vi "Teleop.vi"(10 "Match Info":T1={"Autonomous Elapsed Seconds"=0.0, "TeleOp Elapsed Seconds"=0.0, "Disabled Elapsed Seconds"=0.0, "Visited Autonomous"=FALSE, "Visited TeleOp"=FALSE, "Visited Disabled"=FALSE, "Autonomous Settings"={"Autonomous Style"=enum."Independent", "VI Refnum"=refnum}}, 11 "Call Context":T2) -> ()   [LabVIEW 2019]
doc: "This VI is called for each enabled TeleOp packet received from the DS. It is typically used to read from joysticks and other inputs and update I/O or setpoints for timed control loops. It should complete and return within 20 milliseconds or risk missing DS packets."
uses:
  <vilib>/Rock Robotics/WPI/DriverStation/WPI_DriverStationDerivedRobotMode.ctl
  <vilib>/Rock Robotics/WPI/DriverStation/WPI_DriverStationMatch Info.ctl
  <vilib>/Rock Robotics/WPI/Utilities/WPI_GetSetVariantRefNum.vi
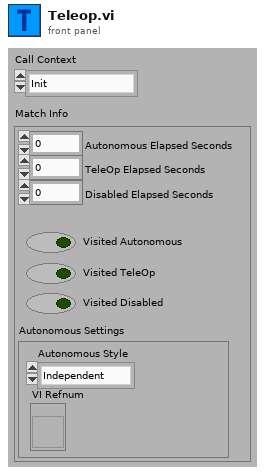
[diagram p1: front panel]
types:
  T1 = typedef "WPI_DriverStationMatch Info.ctl" = cluster{"Autonomous Elapsed Seconds":dbl, "TeleOp Elapsed Seconds":dbl, "Disabled Elapsed Seconds":dbl, "Visited Autonomous":bool, "Visited TeleOp":bool, "Visited Disabled":bool, "Autonomous Settings":cluster{"Autonomous Style":enum16{"Iterative", "Independent"}, "VI Refnum":refnum<vi>}}
  T2 = typedef "WPI_DriverStationDerivedRobotMode.ctl" = enum16{"Init", "Execute", "Stop"}
  T3 = typedef "WPI_JoystickDevRef.ctl" = cluster{"Device":T4}
  T4 = typedef "WPI_JoystickDeviceEnum.ctl" = enum16{"USB 0", "USB 1", "USB 2", "USB 3", "USB 4", "USB 5"}
  T5 = cluster{"POVs[0]":i16, "POVs[1]":i16, "POVs[2]":i16, "POVs[3]":i16, "POVs[4]":i16, "POVs[5]":i16, "POVs[6]":i16, "POVs[7]":i16, "POVs[8]":i16}
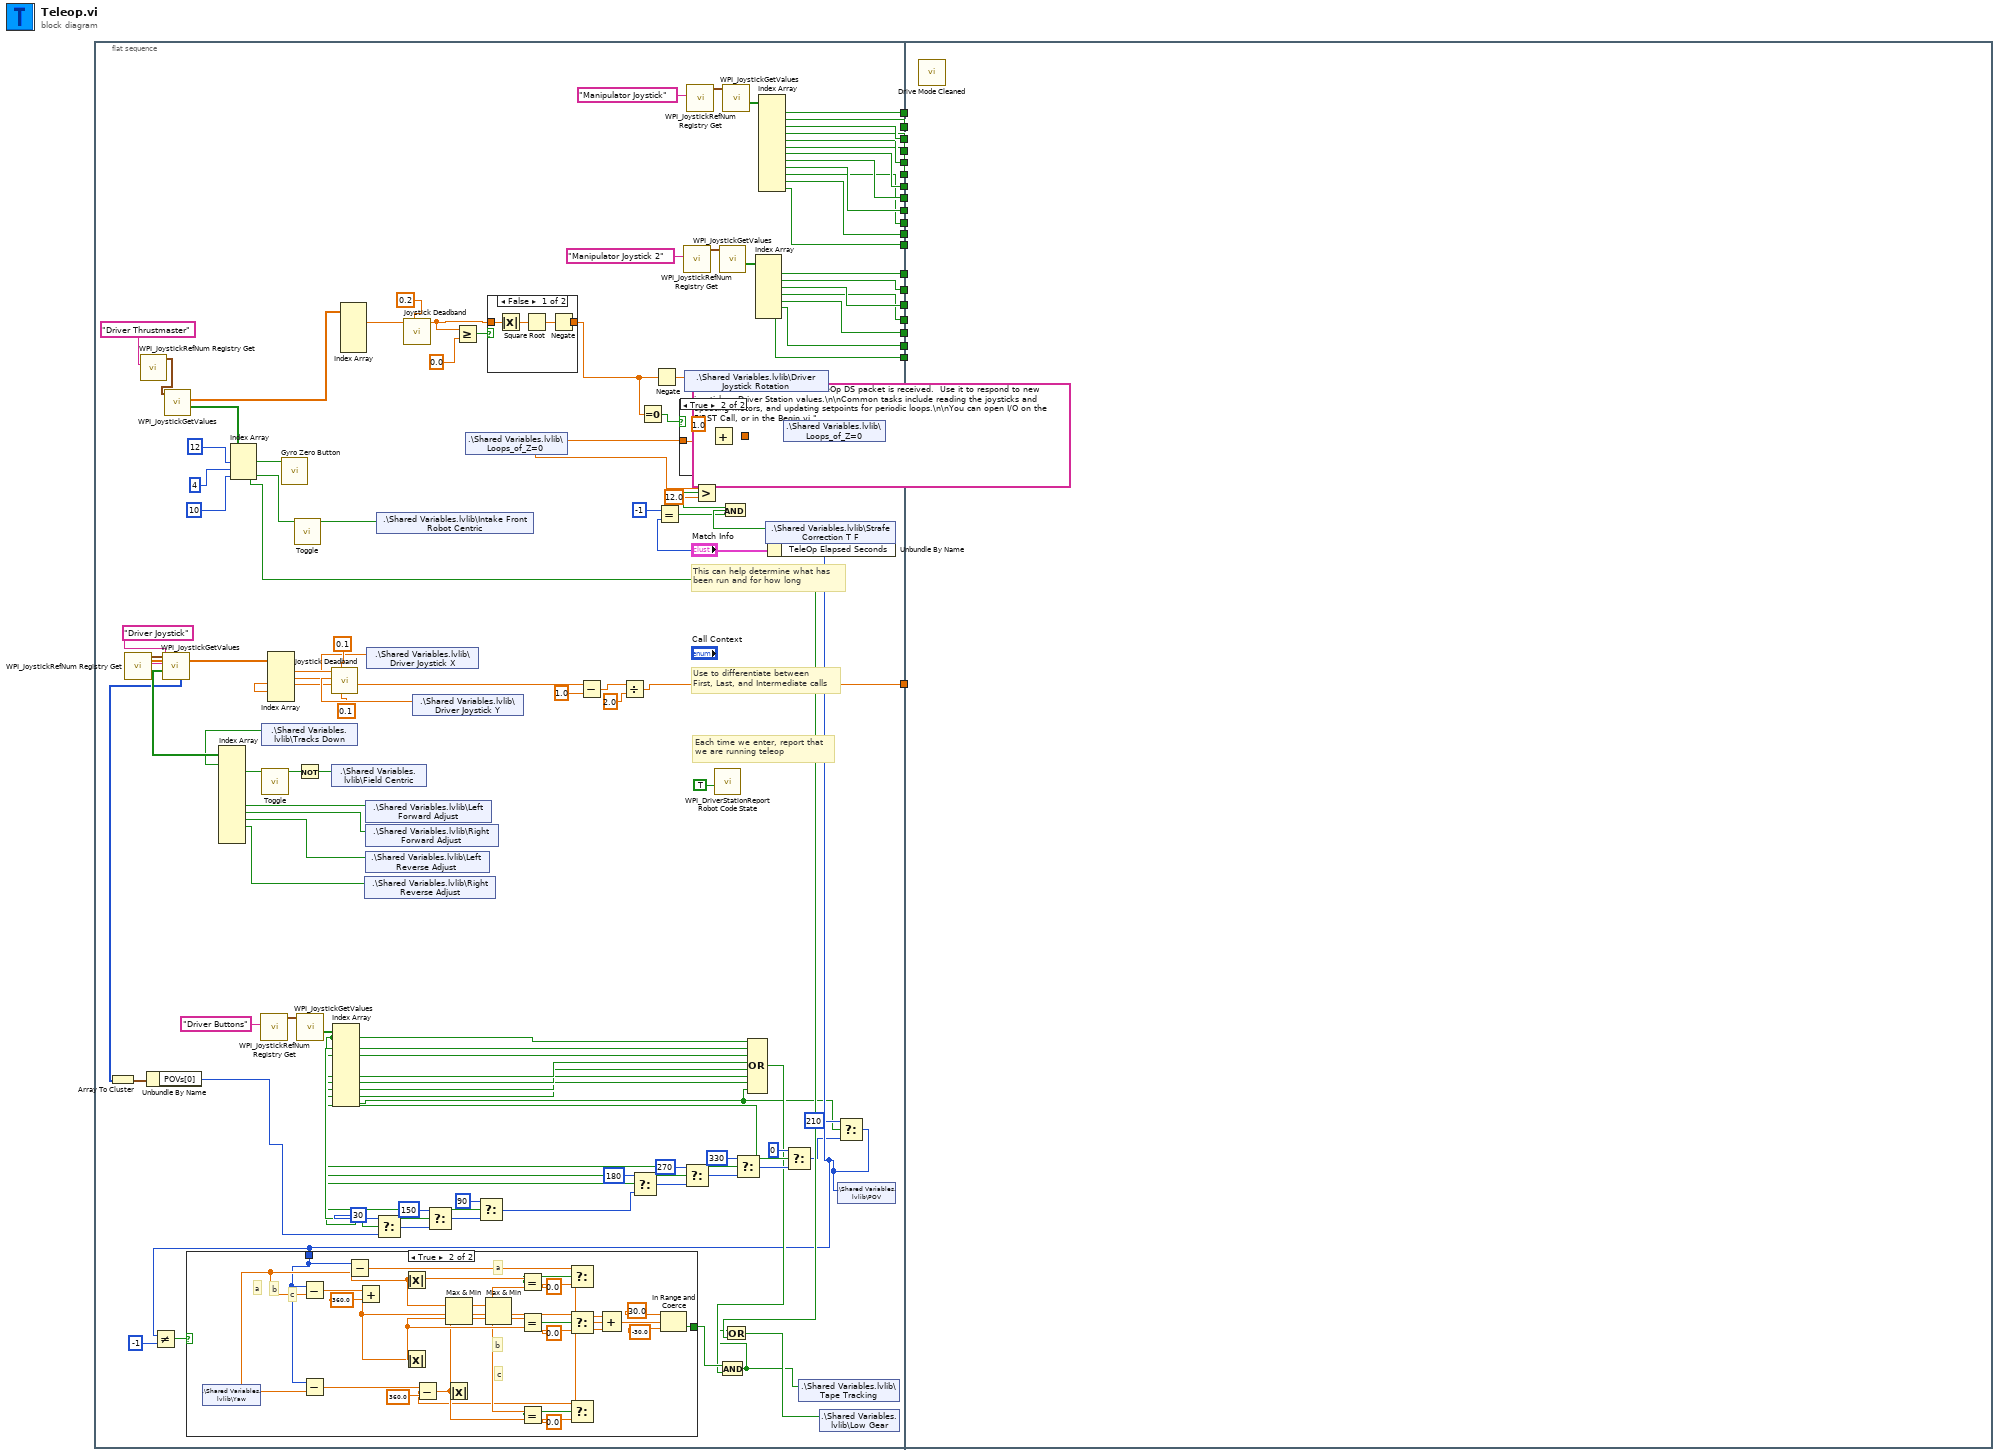
[diagram p0: block diagram]
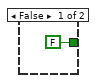
[diagram p2: hidden frame]
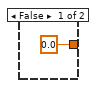
[diagram p3: hidden frame]
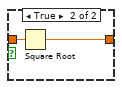
[diagram p4: hidden frame]
diagram:
  (unwired) "This VI is called each time a TeleOp DS packet is received.  Use it to respond to new joystick or Driver Station values.\n\nCommon tasks include reading the joysticks and updating motors, and updating setpoints for periodic loops.\n\nYou can open I/O on the FIRST Call, or in the Begin.vi."
  # "Each time we enter, report that\nwe are running teleop"
  # "Use to differentiate between\nFirst, Last, and Intermediate calls"
  # "This can help determine what has\nbeen run and for how long"
  n1 = flat-sequence {
    tunnel: [w58] -> w20
    tunnel: [w43] -> w19
    tunnel: [w42] -> w18
    tunnel: [w41] -> w17
    tunnel: [w40] -> w16
    tunnel: [w39] -> w15
    tunnel: [w38] -> w14
    tunnel: [w37] -> w13
    tunnel: [w36] -> w12
    tunnel: [w35] -> w11
    tunnel: [w34] -> w10
    tunnel: [w33] -> w9
    tunnel: [w32] -> w8
    tunnel: [w31] -> w7
    tunnel: [w30] -> w6
    tunnel: [w29] -> w5
    tunnel: [w28] -> w4
    tunnel: [w27] -> w3
    tunnel: [w26] -> w2
    tunnel: [w25] -> w1
    tunnel: w20 -> [_]
    tunnel: w19 -> [_]
    tunnel: w18 -> [_]
    tunnel: w17 -> [_]
    tunnel: w16 -> [_]
    tunnel: w15 -> [_]
    tunnel: w14 -> [_]
    tunnel: w13 -> [_]
    tunnel: w12 -> [_]
    tunnel: w11 -> [_]
    tunnel: w10 -> [_]
    tunnel: w9 -> [_]
    tunnel: w8 -> [_]
    tunnel: w7 -> [_]
    tunnel: w6 -> [_]
    tunnel: w5 -> [_]
    tunnel: w4 -> [_]
    tunnel: w3 -> [_]
    tunnel: w2 -> [_]
    tunnel: w1 -> [_]
    frame #0 {
      n2 = call <vilib>:"WPI_JoystickRefNum Registry Get.vi"("refnum name"="Driver Joystick") -> ("JoystickDevRef"=w133:T3)  [unwired: 1 in, 9 out]
      n3 = call <vilib>:"WPI_JoystickRefNum Registry Get.vi"("refnum name"="Driver Thrustmaster") -> ("JoystickDevRef"=w121:T3)  [unwired: 9 in, 1 out]
      n4 = call <vilib>:"WPI_JoystickGetValues.vi"("JoystickDevRef"=w133) -> ("Buttons"=w119:bool[], "Axes"=w131:dbl[], "POVs"=w110:i16[])  [unwired: 6 in, 2 out]
      n5 = Array To Cluster(array=w110) -> (cluster=w111:T5)
      n6 = Unbundle By Name(w111) -> ("POVs[0]"=w44:i16)
      n7 = call <vilib>:"WPI_JoystickGetValues.vi"("JoystickDevRef"=w121) -> ("Buttons"=w116:bool[], "Axes"=w120:dbl[])  [unwired: 6 in, 3 out]
      n8 = Index Array(array=w119) -> (element #1=w98:bool, element #2=w97:bool, element #7=w108:bool, element #8=w107:bool, element #9=w106:bool, element #10=w105:bool)  [unwired: 12 in, 6 out]
      n9 = Index Array(array=w116, index #1=12 ("index"), index #2=4 ("index"), index #3=10 ("index")) -> (element #1=w114:bool, element #2=w62:bool, element #3=w24:bool)
      n10 = call <vilib>:"WPI_JoystickRefNum Registry Get.vi"("refnum name"="Driver Buttons") -> ("JoystickDevRef"=w94:T3)  [unwired: 1 in, 9 out]
      n11 = shared-variable ".\\Shared Variables.lvlib\\Tracks Down"(w98) -> ()  [unwired: 1 in, 1 out]
      n12 = call "Toggle.vi"("Input"=w97) -> ("Output"=w126:bool)  [unwired: 9 in, 1 out]
      n13 = Index Array(array=w131) -> (element #1=w125:dbl, element #2=w124:dbl, element #4=w99:dbl)  [unwired: 5 in, 2 out]
      n14 = call "Gyro Zero Button.vi"("Boolean"=w114) -> ()  [unwired: 11 in]
      n15 = call "Toggle.vi"("Input"=w24) -> ("Output"=w112:bool)  [unwired: 9 in, 1 out]
      n16 = Not(x=w126) -> (.not. x?=w123:bool)
      n17 = call <vilib>:"WPI_JoystickGetValues.vi"("JoystickDevRef"=w94) -> ("Buttons"=w56:bool[])  [unwired: 6 in, 4 out]
      n18 = call "Joystick Deadband.vi"("Z Deadband"=0.1, "X Y Deadband"=0.1, "Z"=w99, "Y"=w124, "X"=w125) -> ("Z Out"=w47:dbl, "Y Out"=w127:dbl, "X Out"=w103:dbl)  [unwired: 4 in]
      n19 = shared-variable ".\\Shared Variables.lvlib\\Field Centric"(w123) -> ()  [unwired: 1 in, 1 out]
      n20 = Index Array(array=w56) -> (element #1=w74:bool, element #2=w80:bool, element #3=w79:bool, element #6=w78:bool, element #7=w77:bool, element #8=w76:bool, element #9=w75:bool, element #10=w48:bool)  [unwired: 10 in, 2 out]
      n21 = Index Array(array=w120) -> (element #1=w102:dbl)  [unwired: 5 in, 4 out]
      n22 = shared-variable ".\\Shared Variables.lvlib\\Right Reverse Adjust"(w105) -> ()  [unwired: 1 in, 1 out]
      n23 = shared-variable ".\\Shared Variables.lvlib\\Left Forward Adjust"(w108) -> ()  [unwired: 1 in, 1 out]
      n24 = shared-variable ".\\Shared Variables.lvlib\\Right Forward Adjust"(w107) -> ()  [unwired: 1 in, 1 out]
      n25 = shared-variable ".\\Shared Variables.lvlib\\Left Reverse Adjust"(w106) -> ()  [unwired: 1 in, 1 out]
      n26 = shared-variable ".\\Shared Variables.lvlib\\Driver Joystick X"(w103) -> ()  [unwired: 1 in, 1 out]
      n27 = Select(t=i16 30, s=w74, f=w44) -> (s? t:f=w88:i16)
      n28 = shared-variable ".\\Shared Variables.lvlib\\Intake Front Robot Centric"(w112) -> ()  [unwired: 1 in, 1 out]
      n29 = call "Joystick Deadband.vi"("X Y Deadband"=0.2, "X"=w102) -> ("X Out"=w100:dbl)  [unwired: 7 in, 2 out]
      n30 = shared-variable ".\\Shared Variables.lvlib\\Driver Joystick Y"(w127) -> ()  [unwired: 1 in, 1 out]
      n31 = Select(t=i16 150, s=w80, f=w88) -> (s? t:f=w87:i16)
      n32 = Greater Or Equal?(x=w100, y=0.0) -> (x >= y?=w118:bool)
      n33 = shared-variable ".\\Shared Variables.lvlib\\Loops_of_Z=0"() -> (w66:dbl)  [unwired: 1 in, 1 out]
      n34 = Select(t=i16 90, s=w79, f=w87) -> (s? t:f=w57:i16)
      n35 = case shown="False" w118 {
        tunnel: [w167 w171] -> w70
        tunnel: w100 -> [w166 w170]
        frame False {
          n36 = Absolute Value(x=w166) -> (abs(x)=w169:dbl)
          n37 = Square Root(x=w169) -> (sqrt(x)=w168:dbl)
          n38 = Negate(x=w168) -> (-x=w167:dbl)
        }
        frame True {
          n39 = Square Root(x=w170) -> (sqrt(x)=w171:dbl)
        }
      }
      n40 = Subtract(x=w47, y=1.0) -> (x-y=w46:dbl)
      n41 = Divide(x=w46, y=2.0) -> (x/y=w58:dbl)
      n42 = Select(t=i16 180, s=w78, f=w57) -> (s? t:f=w85:i16)
      n43 = Equal To 0?(x=w70) -> (x = 0?=w69:bool)
      n44 = Negate(x=w70) -> (-x=w104:dbl)
      n45 = case shown="True" w69 {
        tunnel: w66 -> [_ w165]
        tunnel: [0.0 w163] -> w68
        frame False {
        }
        frame True {
          n46 = Add(x=1.0, y=w165) -> (x+y=w163:dbl)
        }
      }
      n47 = call <vilib>:"WPI_JoystickRefNum Registry Get.vi"("refnum name"="Manipulator Joystick 2") -> ("JoystickDevRef"=w95:T3)  [unwired: 1 in, 9 out]
      n48 = Select(t=i16 270, s=w77, f=w85) -> (s? t:f=w83:i16)
      n49 = shared-variable ".\\Shared Variables.lvlib\\Driver Joystick Rotation"(w104) -> ()  [unwired: 1 in, 1 out]
      n50 = call <vilib>:"WPI_JoystickRefNum Registry Get.vi"("refnum name"="Manipulator Joystick") -> ("JoystickDevRef"=w129:T3)  [unwired: 1 in, 9 out]
      n51 = Greater?(x=w66, y=12.0) -> (0:w67:bool)
      n52 = call <vilib>:"WPI_JoystickGetValues.vi"("JoystickDevRef"=w95) -> ("Buttons"=w54:bool[])  [unwired: 6 in, 4 out]
      n53 = call <vilib>:"WPI_JoystickGetValues.vi"("JoystickDevRef"=w129) -> ("Buttons"=w55:bool[])  [unwired: 6 in, 4 out]
      n54 = Select(t=i16 330, s=w76, f=w83) -> (s? t:f=w81:i16)
      n55 = Compound Arithmetic op=OR(w74, w80, w79, w78, w77, w76, w75, w48) -> (w63:bool)
      n56 = Index Array(array=w54) -> (element #1=w31:bool, element #2=w30:bool, element #3=w29:bool, element #4=w28:bool, element #5=w27:bool, element #6=w26:bool, element #7=w25:bool)  [unwired: 7 in]
      n57 = Index Array(array=w55) -> (element #1=w43:bool, element #2=w42:bool, element #3=w41:bool, element #4=w40:bool, element #5=w39:bool, element #6=w38:bool, element #7=w37:bool, element #8=w36:bool, element #9=w35:bool, element #10=w34:bool, element #11=w33:bool, element #12=w32:bool)  [unwired: 12 in]
      n58 = shared-variable ".\\Shared Variables.lvlib\\Loops_of_Z=0"(w68) -> ()  [unwired: 1 in, 1 out]
      n59 = Select(t=i16 0, s=w75, f=w81) -> (s? t:f=w50:i16)
      n60 = Select(t=i16 210, s=w48, f=w50) -> (s? t:f=w51:i16)
      n61 = Not Equal?(x=w51, y=i16 -1) -> (x != y?=w53:bool)
      n62 = case shown="True" w53 {
        tunnel: [FALSE w159] -> w64
        tunnel: w51 -> [_ w136]
        frame False {
        }
        frame True {
          # "c"
          # "b"
          # "a"
          # "c"
          # "b"
          # "a"
          n63 = shared-variable ".\\Shared Variables.lvlib\\Yaw"() -> (w137:dbl)  [unwired: 1 in, 1 out]
          n64 = Subtract(x=w136, y=w137) -> (x-y=w158:dbl)
          n65 = Subtract(x=w136, y=w137) -> (x-y=w156:dbl)
          n66 = Subtract(x=w136, y=w137) -> (x-y=w147:dbl)
          n67 = Add(x=w158, y=360.0) -> (x+y=w148:dbl)
          n68 = Absolute Value(x=w147) -> (abs(x)=w153:dbl)
          n69 = Absolute Value(x=w148) -> (abs(x)=w152:dbl)
          n70 = Subtract(x=w156, y=360.0) -> (x-y=w146:dbl)
          n71 = Max & Min(x=w153, y=w152) -> (min(x,y)=w154:dbl)  [unwired: 1 out]
          n72 = Absolute Value(x=w146) -> (abs(x)=w150:dbl)
          n73 = Max & Min(x=w154, y=w150) -> (min(x,y)=w151:dbl)  [unwired: 1 out]
          n74 = Equal?(x=w153, y=w151) -> (x = y?=w145:bool)
          n75 = Equal?(x=w151, y=w152) -> (x = y?=w149:bool)
          n76 = Equal?(x=w151, y=w150) -> (x = y?=w144:bool)
          n77 = Select(t=w147, s=w145, f=0.0) -> (s? t:f=w140:dbl)
          n78 = Select(t=w148, s=w149, f=0.0) -> (s? t:f=w139:dbl)
          n79 = Select(t=w146, s=w144, f=0.0) -> (s? t:f=w138:dbl)
          n80 = Compound Arithmetic op=ADD(w140, w139, w138) -> (w135:dbl)
          n81 = In Range and Coerce(upper limit=30.0, x=w135, lower limit=-30.0) -> (In Range?=w159:bool)  [unwired: 1 out]
        }
      }
      n82 = Equal?(x=i16 -1, y=w51) -> (x = y?=w71:bool)
      n83 = And(x=w67, y=w71) -> (x .and. y?=w72:bool)
      n84 = Compound Arithmetic op=AND(w64, w63) -> (w60:bool)
      n85 = Or(x=w60, y=w62) -> (x .or. y?=w61:bool)
      n86 = shared-variable ".\\Shared Variables.lvlib\\Strafe Correction T F"(w72) -> ()  [unwired: 1 in, 1 out]
      n87 = shared-variable ".\\Shared Variables.lvlib\\Tape Tracking"(w60) -> ()  [unwired: 1 in, 1 out]
      n88 = shared-variable ".\\Shared Variables.lvlib\\Low Gear"(w61) -> ()  [unwired: 1 in, 1 out]
      n89 = shared-variable ".\\Shared Variables.lvlib\\POV"(w51) -> ()  [unwired: 1 in, 1 out]
    }
    frame #1 {
      n90 = call "Drive Mode Cleaned.vi"() -> ()  [unwired: 12 in]
    }
  }
  n91 = call <vilib>:"WPI_DriverStationReport Robot Code State.vi"("TeleOp"=TRUE ("Autonomous")) -> ()  [unwired: 10 in, 1 out]
  n92 = Unbundle By Name("Match Info") -> ()  [unwired: 1 out]
